vi "Read stl file, build and save octree.vi"(0 "STL file path (load)":path, 5 "Auto resolution":bool=TRUE, 7 "Specify resolution":sgl=100.0, 9 "Invert model (interior region)":bool, 11 "Octree file path (save)":path) -> (3 "Octree node array":T2[](array[typedef]), 4 "Octree resolution":sgl, 6 "Number of Octree nodes":i32, 8 "Octree branch levels":i32, 10 "Pmax (x, y, z)":sgl[](array[numeric]), 13 "Error out":errorcluster, 14 "Triangles array":T1[](array[typedef]), 15 "Pmin (x, y, z)":sgl[](array[numeric]))   [LabVIEW 2014]
uses:
  Typedefs/TreeNodeBox.ctl
  Typedefs/Quad.ctl
  Typedefs/Quadplane enum.ctl
  Typedefs/Triangle.ctl
panel:
  # "PN 23/01/2015"
  # "Vertices"
  # "Edges"
  # "Unit normal"
  # "Edge unit normals"
  # "Vertices"
  # "Edges"
  # "Unit normal"
  # "Plane ident."
  # "Vertices"
  # "Edges"
  # "Unit normal"
  # "Plane ident."
  # "Vertices"
  # "Edges"
  # "Unit normal"
  # "Plane ident."
  # "Vertices"
  # "Edges"
  # "Unit normal"
  # "Plane ident."
  # "Vertices"
  # "Edges"
  # "Unit normal"
  # "Plane ident."
  # "Vertices"
  # "Edges"
  # "Unit normal"
  # "Plane ident."
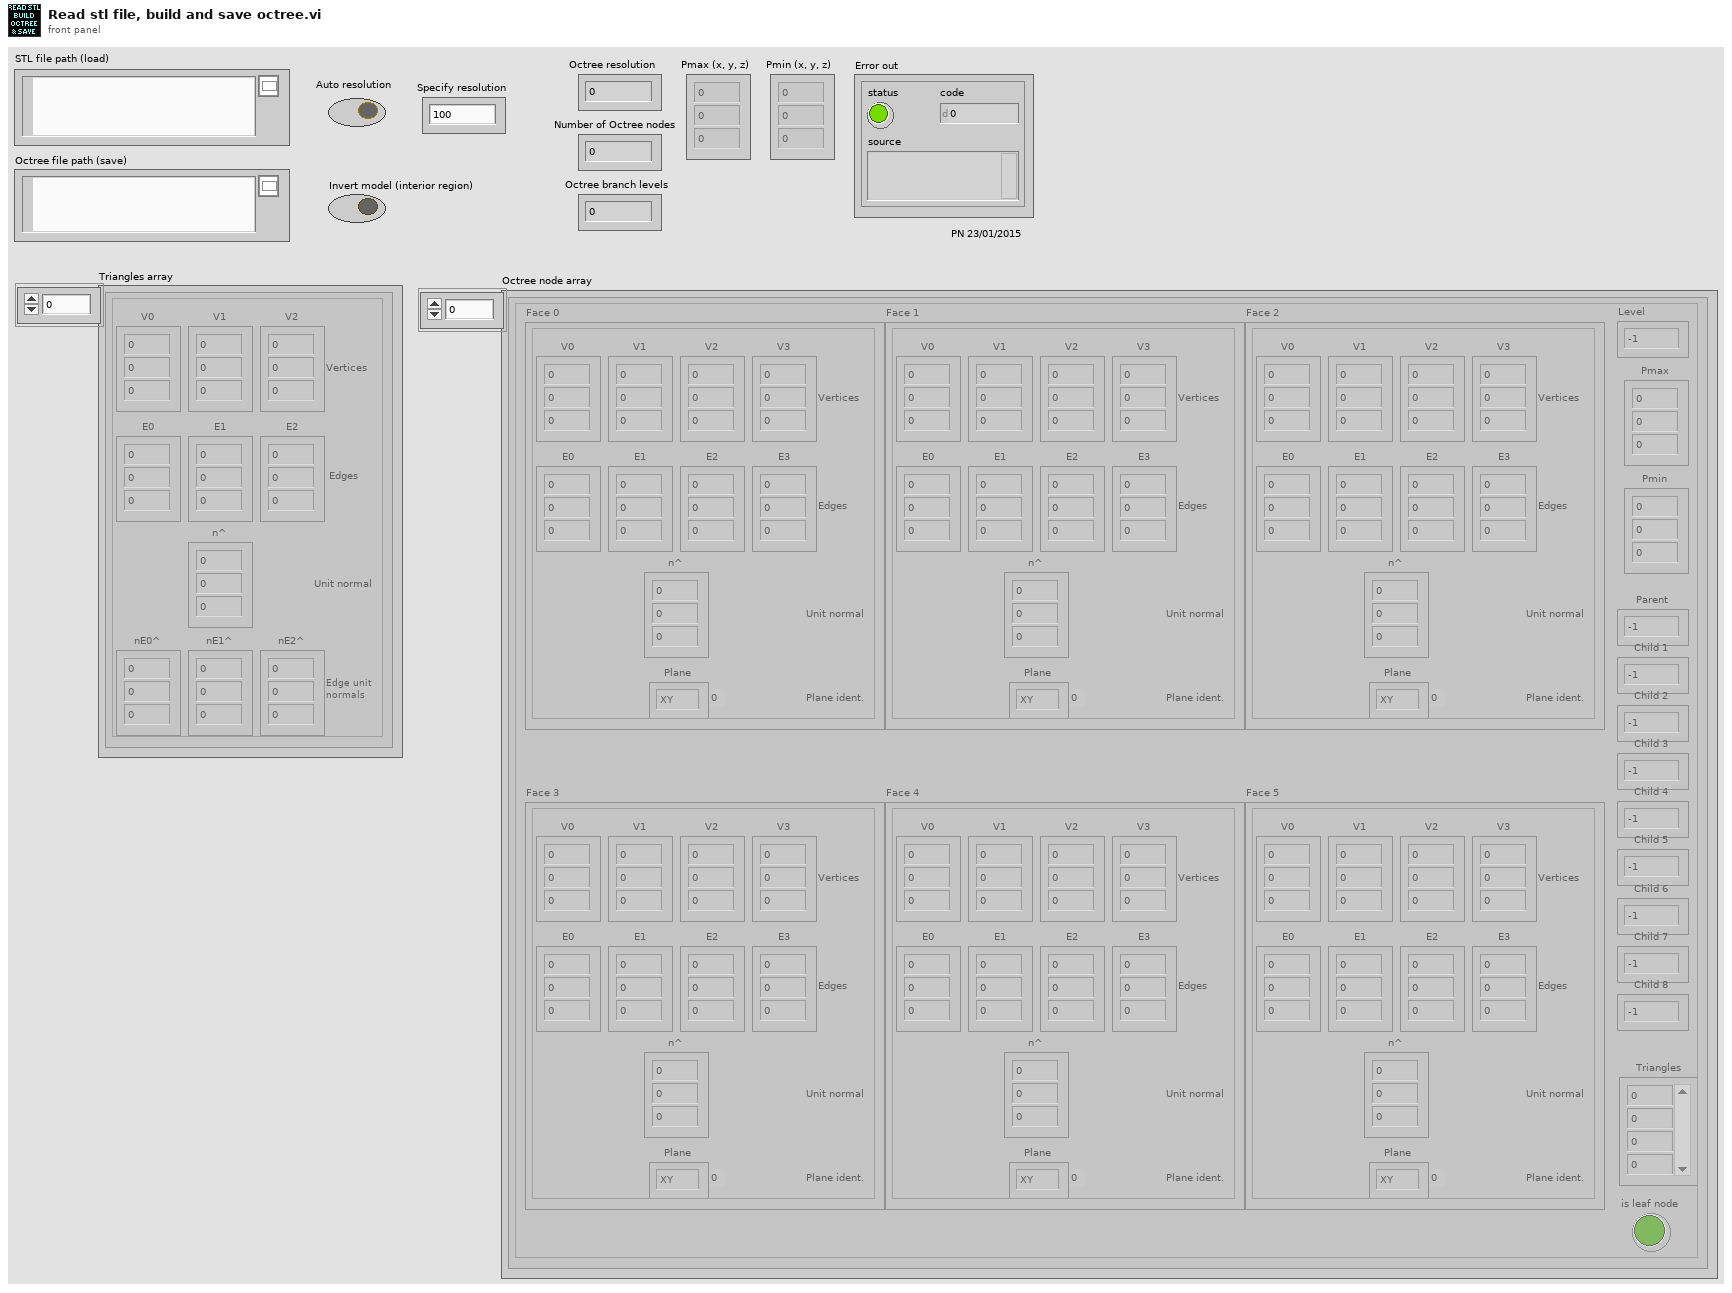
[diagram p1: front panel]
types:
  T1 = typedef "Triangle.ctl" = cluster{"V0":sgl[], "V1":sgl[], "V2":sgl[], "E0":sgl[], "E1":sgl[], "E2":sgl[], "n^":sgl[], "nE0^":sgl[], "nE1^":sgl[], "nE2^":sgl[]}
  T2 = typedef "TreeNodeBox.ctl" = cluster{"Face 0":T3, "Face 1":T3, "Face 2":T3, "Face 3":T3, "Face 4":T3, "Face 5":T3, "Level":i32, "Pmax":sgl[], "Pmin":sgl[], "Parent":i32, "Child 1":i32, "Child 2":i32, "Child 3":i32, "Child 4":i32, "Child 5":i32, "Child 6":i32, "Child 7":i32, "Child 8":i32, "Triangles":i32[], "is leaf node":bool}
  T3 = typedef "Quad.ctl" = cluster{"V0":sgl[], "V1":sgl[], "V2":sgl[], "V3":sgl[], "E0":sgl[], "E1":sgl[], "E2":sgl[], "E3":sgl[], "n^":sgl[], "Plane":T4}
  T4 = typedef "Quadplane enum.ctl" = enum8{"XY", "XZ", "YZ", "-XY", "-XZ", "-YZ"}
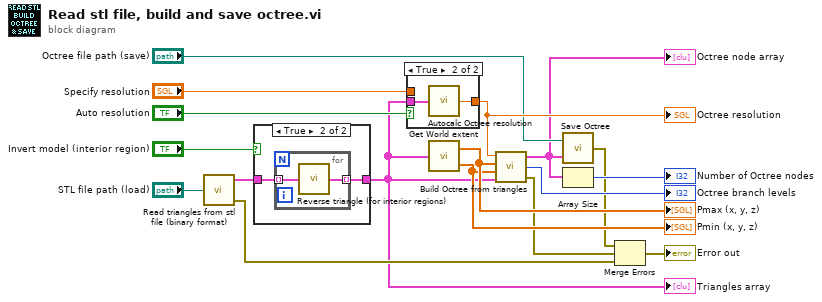
[diagram p0: block diagram]
diagram:
  n1 = call "Read triangles from stl file (binary format).vi"("STL file path"="STL file path (load)") -> ("Triangles array"=w10:T1[], "Error out"=w5:errorcluster)  [unwired: 1 out]
  n2 = case shown="True" "Invert model (interior region)" {
    tunnel: w10 -> [w18 w20]
    tunnel: [w18 w19] -> w1
    frame False {
    }
    frame True {
      n3 = for {
        tunnel: w20 -> [w22] mode=indexing
        tunnel: [w21] -> w19 mode=indexing
        n4 = call "Reverse triangle (for interior regions).vi"("Triangle in"=w22) -> ("Triangle out"=w21:T1)
      }
    }
  }
  "Triangles array" <- w1
  n5 = case shown="True" "Auto resolution" {
    tunnel: [w23 w25] -> w16
    tunnel: w1 -> [_ w24]
    tunnel: "Specify resolution" -> [w23 _]
    frame False {
    }
    frame True {
      n6 = call "Autocalc Octree resolution.vi"("Triangles array"=w24) -> ("Suggested resolution"=w25:sgl)
    }
  }
  "Octree resolution" <- w16
  n7 = call "Get World extent.vi"("Triangles"=w1) -> ("Pmax (x, y, z)"=w14:sgl[], "Pmin (x, y, z)"=w13:sgl[])
  "Pmin (x, y, z)" <- w13
  "Pmax (x, y, z)" <- w14
  n8 = call "Build Octree from triangles.vi"("Triangle array"=w1, "World Pmin (x, y, z)"=w13, "World Pmax (x, y, z)"=w14, "Octree resolution (model units)"=w16) -> ("Stack error"=w4:errorcluster, "Branch levels"=→"Octree branch levels":i32, "Octree node array"=w7:T2[])
  "Octree node array" <- w7
  n9 = call "Save Octree.vi"("Octree node array"=w7, "Octree file path"="Octree file path (save)") -> ("Error out"=w3:errorcluster)
  n10 = Array Size(array=w7) -> (size(s)=→"Number of Octree nodes":i32)
  n11 = Merge Errors(w3, w4, w5) -> (→"Error out":errorcluster)
